vi "Report TPtable.vi"() -> ()   [LabVIEW 2015]
panel:
  out "String":string
  in  "TruePos Input":string[][][](array[string])=[[["F1", "", "", "", "", "", "", ""], ["X", "19.5", "20", "20.5", "20.1", "0.1", "", ""], ["Y", "34.5", "35", "35.5", "34.9", "-0.1", "", ""], ["C3Dia", "9.5", "10", "10.5", "10.213", "0.213", "0.014", ""], ["C1 Dia", "14.5", "15", "15.5", "14.962", "-0.038", "0.007", ""], ["C2Dia", "14.5", "15", "15.5", "15.092", "0.092", "0", ""], ["TP", "0", "MMC", "0.08", "0.07", "0.02", "0.098", "PASS"]], [["F2", "", "", "", "", "", "", ""], ["X", "19.5", "20", "20.5", "20.1", "0.1", "", ""], ["Y", "34.5", "35", "35.5", "34.9", "-0.1", "", ""], ["C3Dia", "9.5", "10", "10.5", "10.213", "0.213", "0.014", ""], ["C1Dia", "14.5", "15", "15.5", "14.962", "-0.038", "0.007", ""], ["C2dia", "14.5", "15", "15.5", "15.092", "0.092", "", ""], ["TP ", "0", "RFS", "0.08", "0.07", "0.02", "0.021", "FAIL"]]]
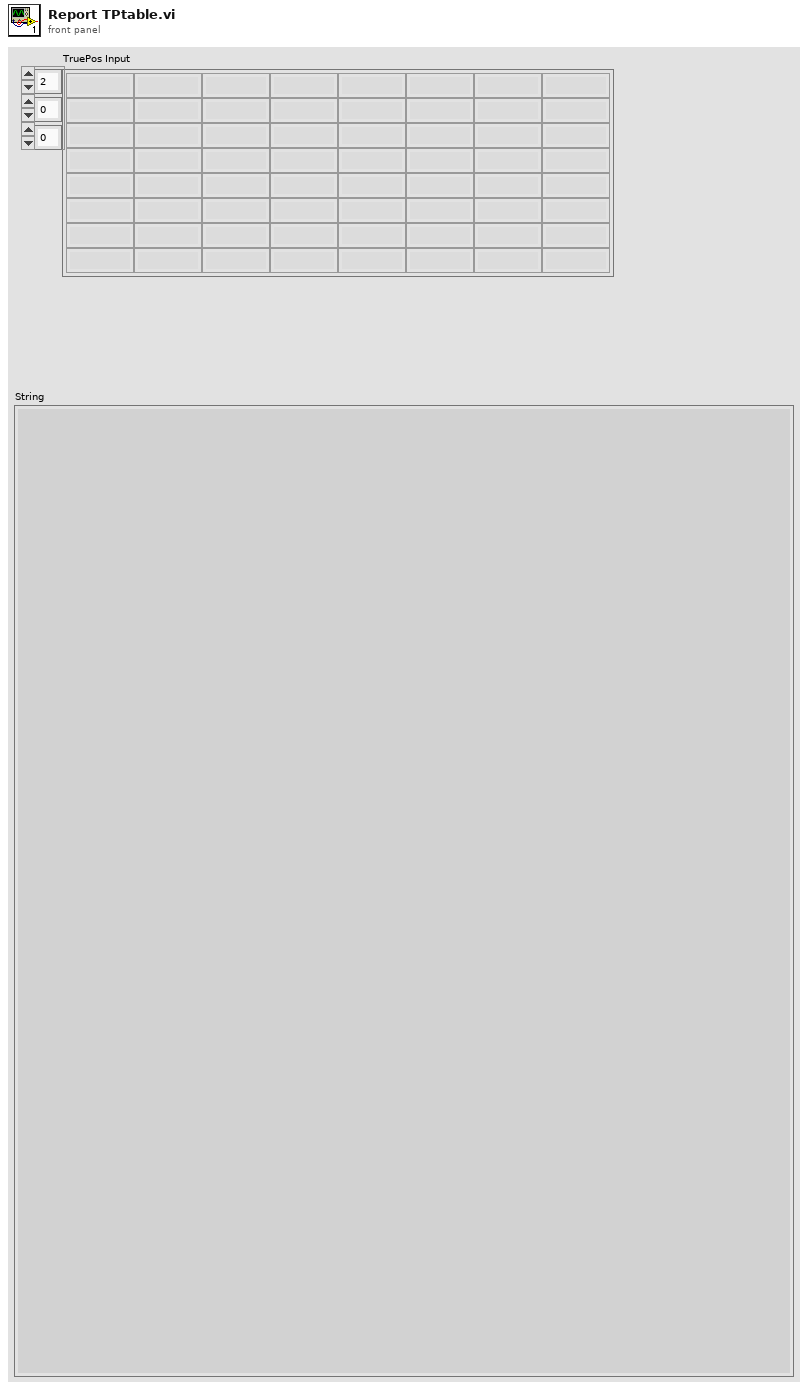
[diagram p1: front panel]
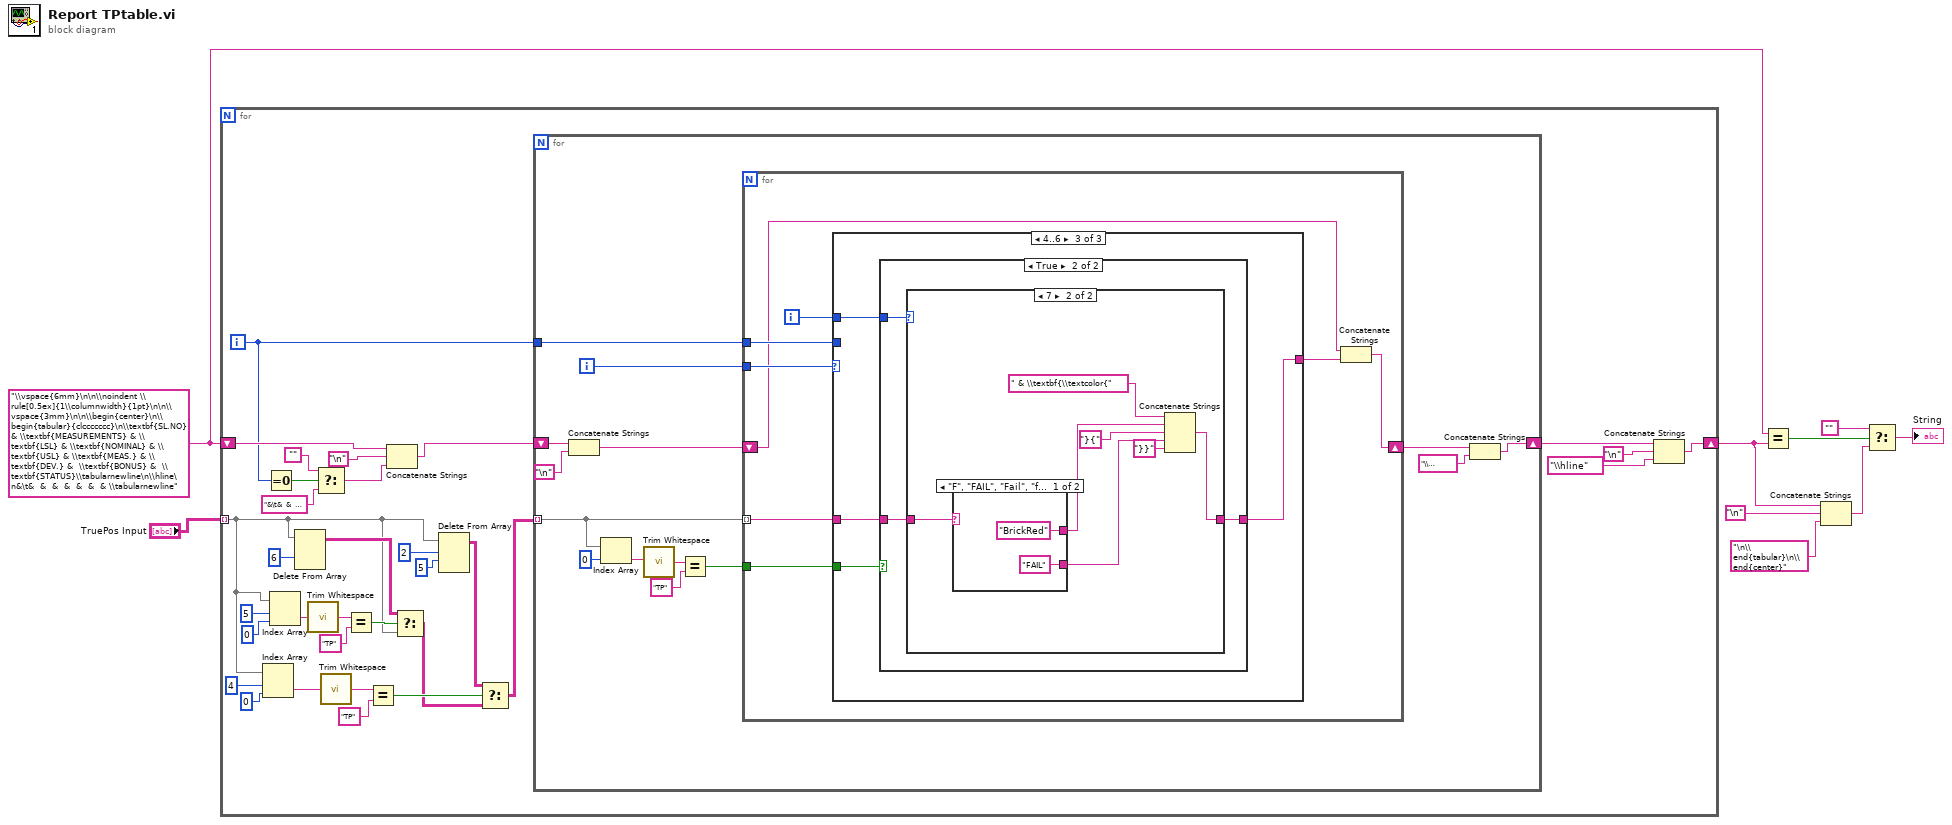
[diagram p0: block diagram]
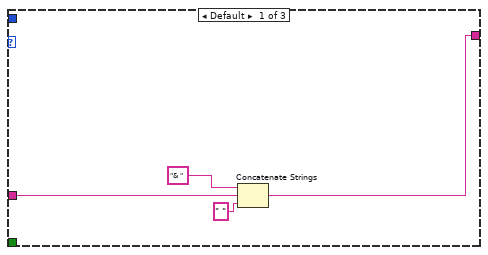
[diagram p2: hidden frame]
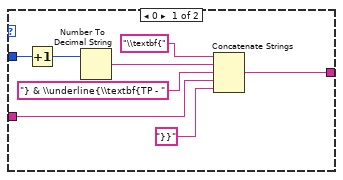
[diagram p4: hidden frame]
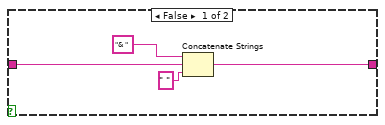
[diagram p5: hidden frame]
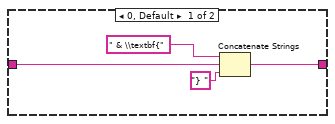
[diagram p6: hidden frame]
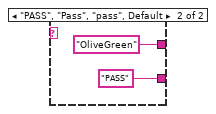
[diagram p7: hidden frame]
diagram:
  w7 = "\\vspace{6mm}\n\n\\noindent \\rule[0.5ex]{1\\columnwidth}{1pt}\n\n\\vspace{3mm}\n\n\\begin{center}\n\\begin{tabular}{clccccccc}\n\\textbf{SL.NO} & \\textbf{MEASUREMENTS} & \\textbf{LSL} & \\textbf{NOMINAL} & \\textbf{USL} & \\textbf{MEAS.} & \\textbf{DEV.} &  \\textbf{BONUS} &  \\textbf{STATUS}\\tabularnewline\n\\hline\n&\t&  &  &  &  &  &  & \\tabularnewline"
  n1 = for {
    tunnel: "TruePos Input" -> [w13] mode=indexing
    shift-right: [w39] -> w5
    shift-left: w7 -> [w36]
    i -> [w34]
    n2 = Index Array(array=w13, index (row)=4, index (col)=0 ("disabled index (col)")) -> (element=w21:string)
    n3 = Equal To 0?(x=w34) -> (x = 0?=w33:bool)
    n4 = Index Array(array=w13, index (row)=5, index (col)=0 ("disabled index (col)")) -> (element=w12:string)
    n5 = Delete From Array(array=w13, index (row)=6) -> (array with subset deleted=w17:string[][])  [unwired: 2 in, 1 out]
    n6 = call <vilib>:"Trim Whitespace.vi"("string"=w12) -> ("trimmed string"=w11:string)  [unwired: 1 in]
    n7 = Select(t="", s=w33, f="&\t&  &  &  &  &  &  & \\tabularnewline") -> (s? t:f=w30:string)
    n8 = call <vilib>:"Trim Whitespace.vi"("string"=w21) -> ("trimmed string"=w10:string)  [unwired: 1 in]
    n9 = Equal?(x=w11, y="TP") -> (x = y?=w19:bool)
    n10 = Equal?(x=w10, y="TP") -> (x = y?=w18:bool)
    n11 = Concatenate Strings(w36, "\n", w30) -> (w35:string)
    n12 = Select(t=w17, s=w19, f=w13) -> (s? t:f=w16:string[][])
    n13 = Delete From Array(array=w13, length=2, index (row)=5) -> (array with subset deleted=w14:string[][])  [unwired: 1 in, 1 out]
    n14 = Select(t=w14, s=w18, f=w16) -> (s? t:f=w15:string[][])
    n15 = for {
      tunnel: w15 -> [w47] mode=indexing
      tunnel: w34 -> [w55]
      shift-right: [w48] -> w41
      shift-left: w35 -> [w53]
      i -> [w54]
      n16 = Concatenate Strings(w53, "\n") -> (w51:string)
      n17 = Index Array(array=w47, index=0) -> (element=w42:string)
      n18 = call <vilib>:"Trim Whitespace.vi"("string"=w42) -> ("trimmed string"=w43:string)  [unwired: 1 in]
      n19 = Equal?(x=w43, y="TP") -> (x = y?=w44:bool)
      n20 = for {
        tunnel: w47 -> [w60] mode=indexing
        tunnel: w55 -> [w61]
        tunnel: w54 -> [w63]
        shift-right: [w57] -> w50
        shift-left: w51 -> [w58]
        tunnel: w44 -> [w56]
        i -> [w62]
        n21 = case shown="4..6" w63 {
          tunnel: w62 -> [_ w71 w84]
          tunnel: w61 -> [_ w70 _]
          tunnel: w60 -> [w66 w69 w83]
          tunnel: [w64 w68 w82] -> w59
          tunnel: w56 -> [_ _ w81]
          frame Default {
            n22 = Concatenate Strings("& " ("string"), w66, " " ("string")) -> (w64:string)
          }
          frame 0 {
            n23 = case shown="Default" w71 {
              tunnel: w70 -> [w79 _]
              tunnel: w69 -> [w75 w80]
              tunnel: [w73 w80] -> w68
              frame 0 {
                n24 = Increment(x=w79) -> (x+1=w72:i32)
                n25 = Number To Decimal String(number=w72) -> (decimal integer string=w77:string)  [unwired: 1 in]
                n26 = Concatenate Strings("\\textbf{" ("string"), w77, "} & \\underline{\\textbf{TP - " ("string"), w75, "}}" ("string")) -> (w73:string)
              }
              frame Default {
              }
            }
          }
          frame 4..6 {
            n27 = case shown="True" w81 {
              tunnel: w84 -> [_ w91]
              tunnel: w83 -> [w86 w90]
              tunnel: [w85 w89] -> w82
              frame False {
                n28 = Concatenate Strings("& " ("string"), w86, " " ("string")) -> (w85:string)
              }
              frame True {
                n29 = case shown="7" w91 {
                  tunnel: w90 -> [w93 w102]
                  tunnel: [w92 w96] -> w89
                  frame 0, Default {
                    n30 = Concatenate Strings(" & \\textbf{" ("string"), w93, "} " ("string")) -> (w92:string)
                  }
                  frame 7 {
                    n31 = case shown="\"F\", \"FAIL\", \"Fail\", \"f\", \"fail\"" w102 {
                      tunnel: ["BrickRed" "OliveGreen"] -> w100
                      tunnel: ["FAIL" "PASS"] -> w98
                      frame "F", "FAIL", "Fail", "f", "fail" {
                      }
                      frame "PASS", "Pass", "pass", Default {
                      }
                    }
                    n32 = Concatenate Strings(" & \\textbf{\\textcolor{", w100, "}{" ("string"), w98, "}}" ("string")) -> (w96:string)
                  }
                }
              }
            }
          }
        }
        n33 = Concatenate Strings(w58, w59) -> (w57:string)
      }
      n34 = Concatenate Strings(w50, "\\tabularnewline" ("string")) -> (w48:string)
    }
    n35 = Concatenate Strings(w41, "\n", "\\hline") -> (w39:string)
  }
  n36 = Equal?(x=w7, y=w5) -> (x = y?=w6:bool)
  n37 = Concatenate Strings(w5, "\n", "\n\\end{tabular}\n\\end{center}") -> (w4:string)
  n38 = Select(t="", s=w6, f=w4) -> (s? t:f=→"String":string)
